vi "Image acquisition color 8-bit RGB - polling.vi"() -> ()   [LabVIEW 2015]
uses:
  C:/code/Host/Installer/Scientific Camera Interfaces/LabVIEW/32_bit/Library_X86/Thorlabs.TSI.TLCameraInterfaces.dll
  code/Host/Installer/Scientific Camera Interfaces/LabVIEW/32_bit/Library_X86/Thorlabs.TSI.TLCameraInterfaces.dll
  SubVIs/Parameters Get & Set/Set Parameters/Set Gain.vi
  SubVIs/Parameters Get & Set/Get Parameters/Get CameraSensorType.vi
  SubVIs/Parameters Get & Set/Get Parameters/Get BitDepth.vi
  SubVIs/Parameters Get & Set/Set Parameters/Set ExposureTime_us.vi
  SubVIs/Parameters Get & Set/Set Parameters/Set FramesPerTrigger_zeroForUnlimited.vi
  SubVIs/Parameters Get & Set/Set Parameters/Set OperationMode.vi
  SubVIs/Parameters Get & Set/Get Parameters/Get NumberOfQueuedFrames.vi
  C:/code/Host/Installer/Scientific Camera Interfaces/LabVIEW/32_bit/Library_X86/Thorlabs.TSI.Demosaicker.dll
  code/Host/Installer/Scientific Camera Interfaces/LabVIEW/32_bit/Library_X86/Thorlabs.TSI.Demosaicker.dll
  C:/code/Host/Installer/Scientific Camera Interfaces/LabVIEW/32_bit/Library_X86/Thorlabs.TSI.ColorProcessor.dll
  code/Host/Installer/Scientific Camera Interfaces/LabVIEW/32_bit/Library_X86/Thorlabs.TSI.ColorProcessor.dll
  C:/code/Host/Installer/Scientific Camera Interfaces/LabVIEW/32_bit/Library_X86/Thorlabs.TSI.ColorInterfaces.dll
  code/Host/Installer/Scientific Camera Interfaces/LabVIEW/32_bit/Library_X86/Thorlabs.TSI.ColorInterfaces.dll
  SubVIs/Color/Color Processor References.ctl
  C:/code/Host/Installer/Scientific Camera Interfaces/LabVIEW/32_bit/Library_X86/Thorlabs.TSI.ImageDataInterfaces.dll
  code/Host/Installer/Scientific Camera Interfaces/LabVIEW/32_bit/Library_X86/Thorlabs.TSI.ImageDataInterfaces.dll
  SubVIs/Parameters Get & Set/Get Parameters/Get ColorFilterArrayPhase.vi
  Controls/Color Balance.ctl
  Controls/Color Modes.ctl
panel:
  in  "Image Type":T1
  in  "Exposure (ms)":u32=100
  in  "Gain":u32 max=1023
  out "new picture":picture
  in  "Color Balance":T2={"Red Gain"=1.0, "Green Gain"=1.0, "Blue Gain"=1.0} {"Blue Gain" min=0 max=10 step=0.05 scale=0.0..10.0 scale format="%#_3g"; "Green Gain" min=0 max=10 step=0.05 scale=0.0..10.0 scale format="%#_3g"; "Red Gain" min=0 max=10 step=0.05 scale=0.0..10.0 scale format="%#_3g"}
  in  "stop":bool
  out "FrameNumber":u32
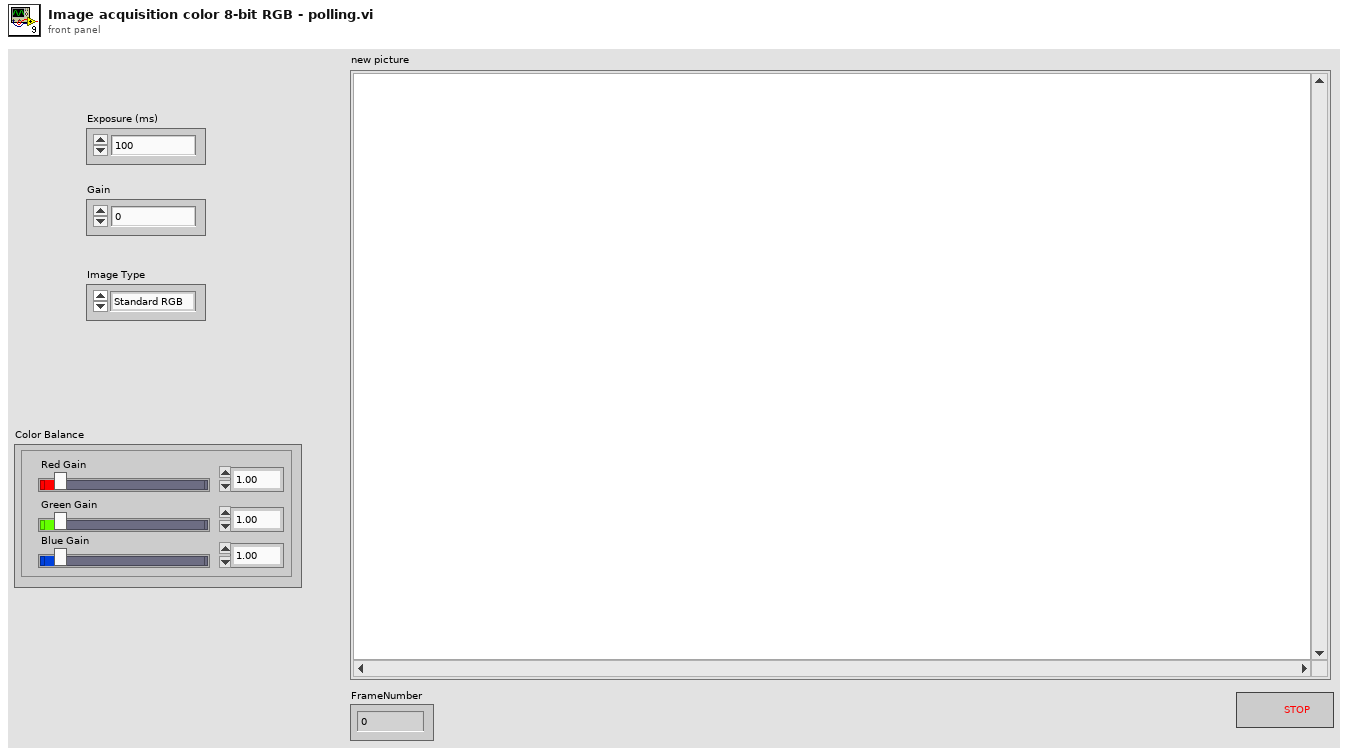
[diagram p1: front panel]
types:
  T1 = typedef "Color Modes.ctl" = enum16{"Standard RGB", "Linear RGB", "Unprocessed"}
  T2 = typedef "Color Balance.ctl" = cluster{"Red Gain":sgl, "Green Gain":sgl, "Blue Gain":sgl}
  T3 = enum8{"Enabled", "Disabled", "Disabled and Grayed Out"}
  T4 = typedef "Color Processor References.ctl" = cluster{"Demosaicker reference":refnum<k24>, "ColorProcessorSDK reference":refnum<k24>, "StandardRGBColorProcessor":refnum<k24>, "LinearRGBColorProcessor":refnum<k24>}
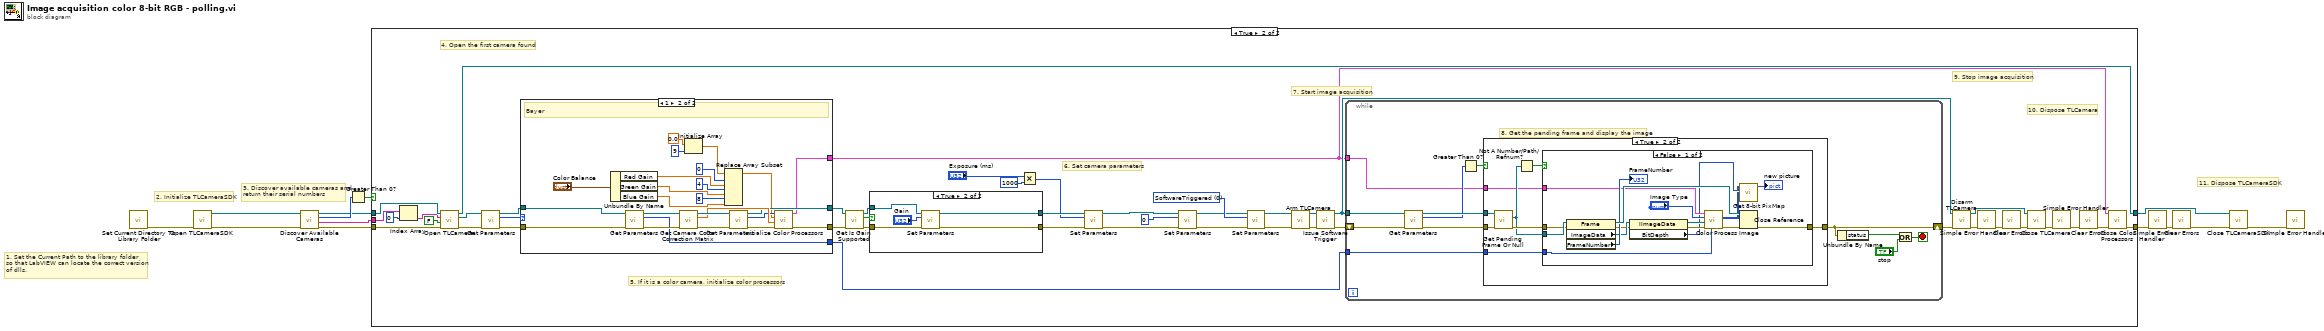
[diagram p0: block diagram]
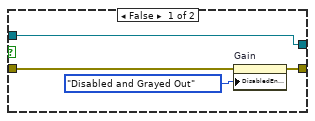
[diagram p3: hidden frame]
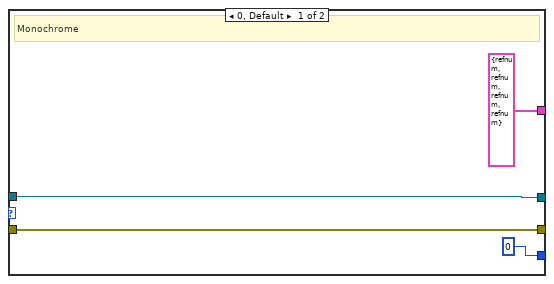
[diagram p4: hidden frame]
diagram:
  # "1. Set the Current Path to the library folder\nso that LabVIEW can locate the correct version\nof dlls."
  # "11. Dispose TLCameraSDK"
  # "3. Discover available cameras and\nreturn their serial numbers"
  # "2. Initialize TLCameraSDK"
  n1 = call "Set Current Directory To Library Folder.vi"() -> ("error out"=w7:errorcluster)  [unwired: 11 in]
  n2 = call "Open TLCameraSDK.vi"("error in (no error)"=w7) -> ("error out"=w6:errorcluster, "TLCameraSDK ref out"=w5:refnum<k24>)  [unwired: 9 in]
  n3 = call "Discover Available Cameras.vi"("error in (no error)"=w6, "TLCameraSDK reference"=w5) -> ("error out"=w11:errorcluster, "Serial Numbers"=w8:string[], "Number of Cameras"=w10:i32, "TLCameraSDK reference out"=w9:refnum<k24>)  [unwired: 6 in]
  n4 = Greater Than 0?(x=w10) -> (x > 0?=w12:bool)
  n5 = case shown="True" w12 {
    tunnel: w9 -> [w14 w60]
    tunnel: w11 -> [w15 w43]
    tunnel: [w15 w22] -> w1
    tunnel: [w14 w57] -> w13
    tunnel: w8 -> [_ w55]
    frame False {
    }
    frame True {
      w32 = 0 items=["SoftwareTriggered", "HardwareTriggered", "Bulb", "Reserved1", "Reserved2"] ("OperationMode")
      # "10. Dispose TLCamera"
      # "9. Stop image acquisition"
      # "7. Start image acquisition"
      # "6. Set camera parameters"
      # "5. If it is a color camera, initialize color processors"
      # "4. Open the first camera found"
      n6 = Index Array(array=w55, index=0) -> (element=w42:string)
      n7 = call "Open TLCamera.vi"("error in (no error)"=w43, "isDiagnosticsMessagesEnabled"=FALSE, "Camera serial number"=w42, "TLCameraSDK reference"=w60) -> ("error out"=w40:errorcluster, "TLCamera reference out"=w41:refnum<k24>, "TLCameraSDK reference out"=w57:refnum<k24>)  [unwired: 5 in]
      n8 = call-poly "Get Parameters.vi"("error in (no error)"=w40, "TLCamera reference in"=w41) -> ("error out"=w39:errorcluster, "CameraSensorType"=w38:i32, "TLCamera reference out"=w54:refnum<k24>)  [unwired: 7 in]
      n9 = case shown="1" w38 {
        tunnel: w54 -> [w72 w78]
        tunnel: w39 -> [w73 w77]
        tunnel: [w73 w82] -> w45
        tunnel: [w72 w83] -> w46
        tunnel: [T4 {"Demosaicker reference"=refnum, "ColorProcessorSDK reference"=refnum, "StandardRGBColorProcessor"=refnum, "LinearRGBColorProcessor"=refnum} ("Color Processor References") w81] -> w21
        tunnel: [0 ("ColorFilterArrayPhase") w74] -> w16
        frame 0, Default {
          # "Monochrome"
        }
        frame 1 {
          # "Bayer"
          n10 = Unbundle By Name("Color Balance") -> ("Red Gain"=w93:sgl, "Green Gain"=w95:sgl, "Blue Gain"=w97:sgl)
          n11 = call-poly "Get Parameters.vi"("error in (no error)"=w77, "TLCamera reference in"=w78) -> ("error out"=w75:errorcluster, "ColorFilterArrayPhase"=w74:i32, "TLCamera reference out"=w76:refnum<k24>)  [unwired: 7 in]
          n12 = call "Get Camera Color Correction Matrix.vi"("error in (no error)"=w75, "TLCamera reference"=w76) -> ("error out"=w87:errorcluster, "Camera Color Correction Matrix"=w84:sgl[], "TLCamera reference out"=w86:refnum<k24>)  [unwired: 7 in]
          n13 = Initialize Array(sgl 0.0 ("element"), 9 ("dimension size")) -> (w90:sgl[])
          n14 = Replace Array Subset(array=w90, new element #1=w93, index #1=0 ("index"), new element #2=w95, index #2=4 ("index"), new element #3=w97, index #3=8 ("index")) -> (w79:sgl[])
          n15 = call-poly "Get Parameters.vi"("error in (no error)"=w87, "TLCamera reference in"=w86) -> ("error out"=w85:errorcluster, "BitDepth"=w80:u32, "TLCamera reference out"=w83:refnum<k24>)  [unwired: 7 in]
          n16 = call "Initialize Color Processors.vi"("error in (no error)"=w85, "Camera Color Correction Matrix"=w84, "White Balance Matrix"=w79, "BitDepth"=w80) -> ("error out"=w82:errorcluster, "Color Processor References"=w81:T4)  [unwired: 6 in]
        }
      }
      n17 = call "Get Is Gain Supported.vi"("error in (no error)"=w45, "TLCamera reference in"=w46) -> ("error out"=w47:errorcluster, "Is Gain Supported?"=w49:bool, "TLCamera reference out"=w48:refnum<k24>)  [unwired: 7 in]
      n18 = case shown="True" w49 {
        tunnel: w48 -> [w61 w67]
        tunnel: w47 -> [w62 w69]
        tunnel: [w63 w68] -> w36
        tunnel: [w61 w66] -> w44
        frame False {
          n19 = property on="Gain" class="DigNum (strict)"(error in=w62, "DisabledEnum"=T3."Disabled and Grayed Out" ("Disabled")) -> (error out=w63:errorcluster)  [unwired: 1 in, 1 out]
        }
        frame True {
          n20 = call-poly "Set Parameters.vi"("error in (no error)"=w69, "Gain"="Gain", "TLCamera reference in"=w67) -> ("error out"=w68:errorcluster, "TLCamera reference out"=w66:refnum<k24>)  [unwired: 7 in]
        }
      }
      n21 = Multiply(x="Exposure (ms)", y=u32 1000) -> (x*y=w37:u32)
      n22 = call-poly "Set Parameters.vi"("error in (no error)"=w36, "ExposureTime_us"=w37, "TLCamera reference in"=w44) -> ("error out"=w33:errorcluster, "TLCamera reference out"=w34:refnum<k24>)  [unwired: 7 in]
      n23 = call-poly "Set Parameters.vi"("error in (no error)"=w33, "FramesPerTrigger_zeroForUnlimited"=u32 0 ("FramesPerTriggerOrZeroForUnlimited"), "TLCamera reference in"=w34) -> ("error out"=w30:errorcluster, "TLCamera reference out"=w31:refnum<k24>)  [unwired: 7 in]
      n24 = call-poly "Set Parameters.vi"("error in (no error)"=w30, "OperationMode"=w32, "TLCamera reference in"=w31) -> ("error out"=w17:errorcluster, "TLCamera reference out"=w18:refnum<k24>)  [unwired: 7 in]
      n25 = call "Arm TLCamera.vi"("error in (no error)"=w17, "TLCamera reference"=w18) -> ("error out"=w19:errorcluster, "TLCamera reference out"=w20:refnum<k24>)  [unwired: 8 in]
      n26 = call "Issue Software Trigger.vi"("error in (no error)"=w19, "TLCamera Reference"=w20) -> ("error out"=w52:errorcluster, "TLCamera reference out"=w53:refnum<k24>)  [unwired: 8 in]
      n27 = while {
        tunnel: w53 -> [w109]
        shift-right: [w106] -> w29
        shift-left: w52 -> [w102]
        tunnel: w21 -> [w99]
        tunnel: w16 -> [w98]
        stop <- w103 stop-if-true
        # "8. Get the pending frame and display the image"
        n28 = call-poly "Get Parameters.vi"("error in (no error)"=w102, "TLCamera reference in"=w109) -> ("error out"=w100:errorcluster, "NumberOfQueuedFrames"=w101:i32, "TLCamera reference out"=w107:refnum<k24>)  [unwired: 7 in]
        n29 = Greater Than 0?(x=w101) -> (x > 0?=w108:bool)
        n30 = case shown="True" w108 {
          tunnel: w100 -> [w110 w115]
          tunnel: w107 -> [_ w118]
          tunnel: [w110 w116] -> w106
          tunnel: w99 -> [_ w112]
          tunnel: w98 -> [_ w111]
          frame False {
          }
          frame True {
            n31 = call "Get Pending Frame Or Null.vi"("error in (no error)"=w115, "TLCamera reference"=w118) -> ("error out"=w114:errorcluster, "Pending Frame Or Null"=w113:refnum<k24>)  [unwired: 7 in, 1 out]
            n32 = Not A Number/Path/Refnum?(number/path/refnum=w113) -> (NaN/Path/Refnum?=w117:bool)
            n33 = case shown="False" w117 {
              tunnel: w113 -> [w134 _]
              tunnel: w114 -> [w133 w135]
              tunnel: [w131 w135] -> w116
              tunnel: w112 -> [w128 _]
              tunnel: w111 -> [w126 _]
              frame False {
                n34 = property class="Frame"(reference=w134, error in=w133) -> (reference out=w132:refnum<k24>, error out=w123:errorcluster, "ImageData"=w125:refnum<k24>, "FrameNumber"=→"FrameNumber":u32)
                n35 = property class="IImageData"(reference=w125, error in=w123) -> (reference out=w124:refnum<k24>, error out=w122:errorcluster, "BitDepth"=w120:i32)
                n36 = call "Color Process Image.vi"("Color Filter Array Phase"=w126, "error in (no error)"=w122, "ImageData"=w124, "Image Type"="Image Type", "Color Processor References"=w128) -> ("error out"=w121:errorcluster, "Color Data"=w119:u16[][][])  [unwired: 5 in]
                n37 = call "Get 8-bit PixMap.vi"("Original Bit depth"=w120, "Color Data"=w119) -> ("new picture"=→"new picture":picture)  [unwired: 9 in]
                n38 = Close Reference(reference=w132, error in (no error)=w121) -> (error out=w131:errorcluster)
              }
              frame True {
              }
            }
          }
        }
        n39 = Unbundle By Name(w106) -> ("status"=w105:bool)
        n40 = Or(x=w105, y="stop") -> (x .or. y?=w103:bool)
      }
      n41 = call "Disarm TLCamera.vi"("error in (no error)"=w29, "TLCamera reference"=w53) -> ("error out"=w28:errorcluster, "TLCamera reference out"=w58:refnum<k24>)  [unwired: 8 in]
      n42 = call <vilib>:"Simple Error Handler.vi"("error in (no error)"=w28) -> ("error out"=w27:errorcluster)  [unwired: 4 in, 4 out]
      n43 = call <vilib>:"Clear Errors.vi"("error in (no error)"=w27) -> ("error out"=w26:errorcluster)  [unwired: 5 in, 1 out]
      n44 = call "Close TLCamera.vi"("error in (no error)"=w26, "TLCamera reference"=w58) -> ("error out"=w24:errorcluster)  [unwired: 9 in]
      n45 = call <vilib>:"Simple Error Handler.vi"("error in (no error)"=w24) -> ("error out"=w25:errorcluster)  [unwired: 4 in, 4 out]
      n46 = call <vilib>:"Clear Errors.vi"("error in (no error)"=w25) -> ("error out"=w23:errorcluster)  [unwired: 5 in, 1 out]
      n47 = call "Close Color Processors.vi"("error in (no error)"=w23, "Color Processor References"=w21) -> ("error out"=w22:errorcluster)  [unwired: 9 in]
    }
  }
  n48 = call <vilib>:"Simple Error Handler.vi"("error in (no error)"=w1) -> ("error out"=w3:errorcluster)  [unwired: 4 in, 4 out]
  n49 = call <vilib>:"Clear Errors.vi"("error in (no error)"=w3) -> ("error out"=w2:errorcluster)  [unwired: 5 in, 1 out]
  n50 = call "Close TLCameraSDK.vi"("error in (no error)"=w2, "TLCameraSDK reference"=w13) -> ("error out"=w4:errorcluster)  [unwired: 9 in]
  n51 = call <vilib>:"Simple Error Handler.vi"("error in (no error)"=w4) -> ()  [unwired: 4 in, 5 out]
